vi "Read Amplitude.vi"(8 "error in (no error)":errorcluster, 11 "Function Generator in":refnum<class "Function Generator.lvclass">) -> (0 "error out":errorcluster, 2 "Amplitude":dbl[unit], 3 "Function Generator out":refnum<class "Function Generator.lvclass">)   [LabVIEW 2023, in "Function Generator.lvclass"]
uses:
  Function Generator.lvclass
  Function Generator.lvclass/Function Generator.ctl
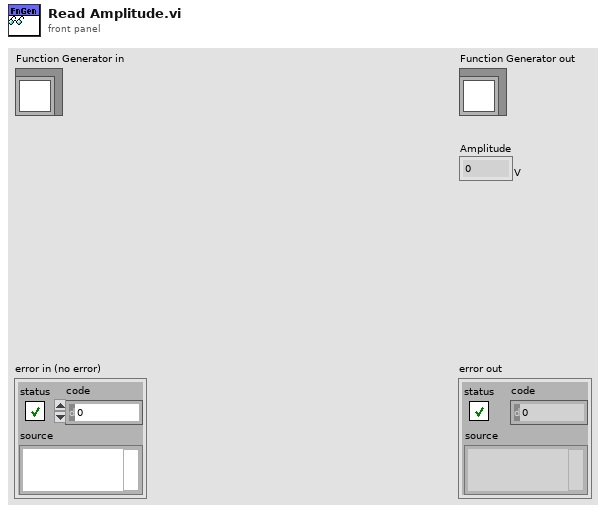
[diagram p1: front panel]
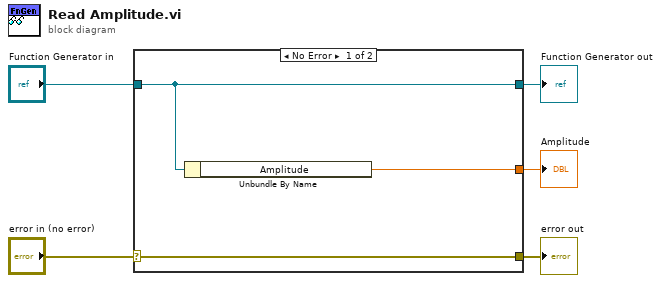
[diagram p0: block diagram]
diagram:
  n1 = case shown="No Error" "error in (no error)" {
    selector: "error in (no error)" -> [w8 w9]
    tunnel: [w8 w9] -> w4
    tunnel: [w7 w10] -> w2
    tunnel: "Function Generator in" -> [w7 w10]
    tunnel: [w6 _] -> w1
    frame No Error {
      n2 = Unbundle By Name(w7) -> ("Amplitude"=w6:dbl[unit])
    }
    frame Error {
    }
  }
  "error out" <- w4
  "Function Generator out" <- w2
  "Amplitude" <- w1
